vi "Shutdown HW.vi"(8 "error in (no error)":errorcluster, 11 "Simulated Camera in":refnum<class "Simulated Camera.lvclass">) -> (0 "error out":errorcluster, 3 "Simulated Camera out":refnum<class "Simulated Camera.lvclass">)   [LabVIEW 2020, in "Simulated Camera.lvclass"]
uses:
  Simulated Camera.lvclass
  Camera.lvclass
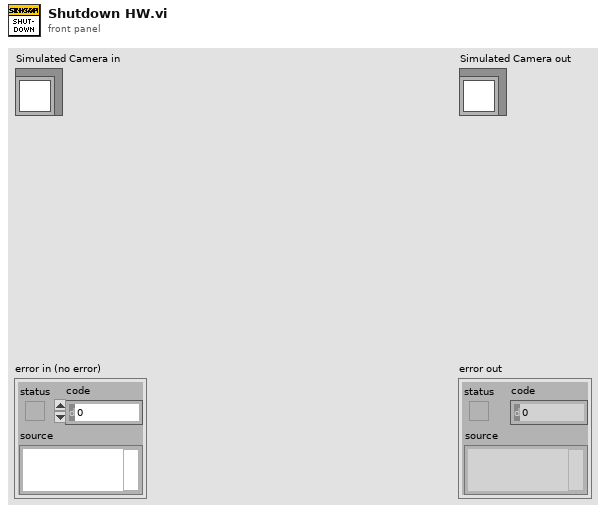
[diagram p1: front panel]
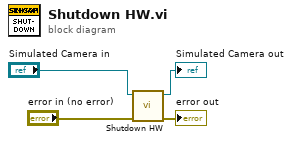
[diagram p0: block diagram]
diagram:
  n1 = call-parent "Shutdown HW.vi"("error in (no error)"="error in (no error)", "Camera in"="Simulated Camera in") -> ("error out"=→"error out":errorcluster, "Camera out"=→"Simulated Camera out":refnum<class "Simulated Camera.lvclass">)  [unwired: 8 in]
